vi "Check Plugin Active.vi"(8 "error in (no error)":errorcluster, 10 "Plugin":string, 11 "Execution UI in":refnum<class "Execution UI.lvclass">) -> (0 "error out":errorcluster, 2 "Active?":bool, 3 "Execution UI out":refnum<class "Execution UI.lvclass">)   [LabVIEW 2020, in "Execution UI.lvclass"]
uses:
  Execution UI.lvclass
  Execution UI.lvclass/Execution UI.ctl
  Framework/Plugin/Plugin.lvclass
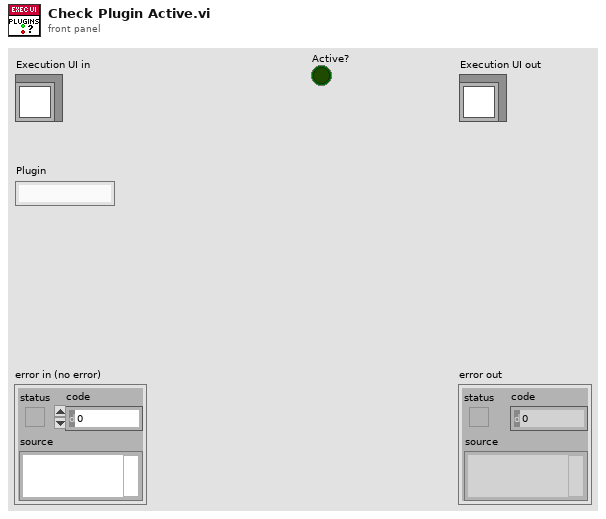
[diagram p1: front panel]
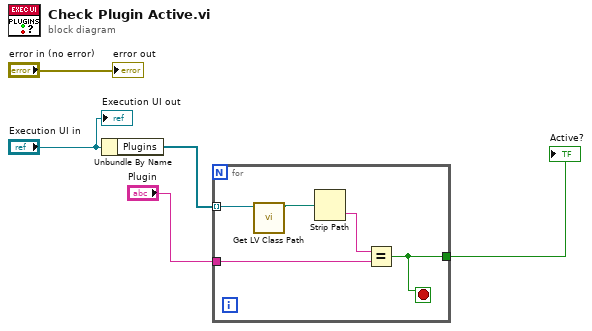
[diagram p0: block diagram]
diagram:
  n1 = Unbundle By Name("Execution UI in") -> ("Plugins"=w3:refnum<class "Plugin.lvclass">[])
  n2 = for {
    tunnel: w3 -> [w10] mode=indexing
    tunnel: "Plugin" -> [w7]
    tunnel: [w6] -> w1
    stop <- w6 stop-if-true
    n3 = call <vilib>:"Get LV Class Path.vi"("object"=w10) -> ("class path"=w9:path)  [unwired: 9 in, 1 out]
    n4 = Strip Path(path=w9) -> (name=w8:string)  [unwired: 1 out]
    n5 = Equal?(x=w8, y=w7) -> (x = y?=w6:bool)
  }
  "Active?" <- w1
  "error out" <- "error in (no error)"
  "Execution UI out" <- "Execution UI in"
